vi "New Verify as JSON.vi"   [LabVIEW 2020, in "Caraya.Extension.lvlib"]
uses:
  Caraya.Extension.lvlib
  <vilib>/addons/_JKI Toolkits/Caraya/classes/Test/Test.lvclass
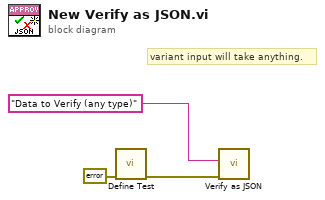
[diagram p0: block diagram]
diagram:
  # "variant input will take anything."
  n1 = call <vilib>:"Define Test.vi"("error in (no error)"=errorcluster {"status"=FALSE, "code"=0, "source"=""}) -> ("error out"=w2:errorcluster)  [unwired: 9 in, 1 out]
  n2 = call "Verify as JSON.vi"("error in"=w2, "Anything"="Data to Verify (any type)") -> ()  [unwired: 8 in, 2 out]
